vi "WT300 IEC 2015 Setup.vi"(0 "VISA Input":refnum<visa-resource-name>="WT210", 5 "Update Rate (250m s)":dbl(ring)=0.1 format="%#_13g" items=["100m"=0.1, "250m"=0.25, "500m"=0.5, "1"=1.0, "2"=2.0, "5"=5.0], 7 "Range Configuration (True)":bool[](array[boolean])=[FALSE, FALSE, FALSE, FALSE, FALSE, FALSE, FALSE, TRUE, TRUE, TRUE, TRUE, TRUE, FALSE], 11 "error in (no error)":errorcluster, 12 "Enable Auto Range (F: Disable)":bool, 13 "Manual Range (20 <10> A)":dbl(ring)=10.0 items=["5m <2.5m>"=0.0025, "10m <5m>"=0.005, "20m <10m>"=0.01, "50m <25m>"=0.025, "100m <50m>"=0.05, "200m <100m>"=0.1, "500m <250m>"=0.25, "1 <500m>"=0.5, "2 <1>"=1.0, "5 <2.5>"=2.5, "10 <5>"=5.0, "20 <10>"=10.0, "40 <20>"=20.0]) -> (2 "VTHD":sgl=0.065 format="%.3g", 4 "VISA Output":refnum<visa-resource-name>="WT210", 6 "Header File":string[][](array[string])=[["Instrument", "YOKOGAWA,WT332,C2QB17128V,F1.03\n"], ["Instr Driver Revision", "1.0 F1.03"], ["Start Time", "1.0"], ["Voltage Range", "6/1/2015 11:50 AM"], ["Current Range", "Auto"], ["Update Rate", "Auto"], ["Standard", "0.250"], ["Algorithm", "IEC62301 Ed.2(Auto)"], ["Stop Factor", "Linear Regression"], ["Valid Period", ""], ["Start Total Harmonic Distortion Uthd 1", "0.065"], ["Start Total Harmonic Distortion Uthd 2", ""], ["End Total Harmonic Distortion Uthd 1", ""], ["End Total Harmonic Distortion Uthd 2", ""], ["Max Power (Watts)", ""], ["Power Variation (%)", ""], ["", ""]], 15 "error out":errorcluster)   [LabVIEW 2016]
uses:
  <vilib>/Utility/error.llb/whitespace.ctl
  Public/Utility/Function/Create Function String (Harmonics).vi
  Public/Data/Read Measurement (Normal).vi
  Yokogawa WT300 Series.lvlib
panel:
  out "Date & Time":string="6/1/2015 11:50 AM"
  out "Instrument ID":string="YOKOGAWA,WT332,C2QB17128V,F1.03\n"
  out "Sample Rate":string="0.250"
  # "5m <2.5m> A"
  # "10m <5m> A"
  # "20m <10m> A"
  # "50m <25m> A"
  # "100m <50m> A"
  # "200m <100m> A"
  # "500m <250m> A"
  # "1 <500m> A"
  # "2 <1> A"
  # "5 <2.5> A"
  # "10 <5> A"
  # "20 <10> A"
  # "40 <20> A"
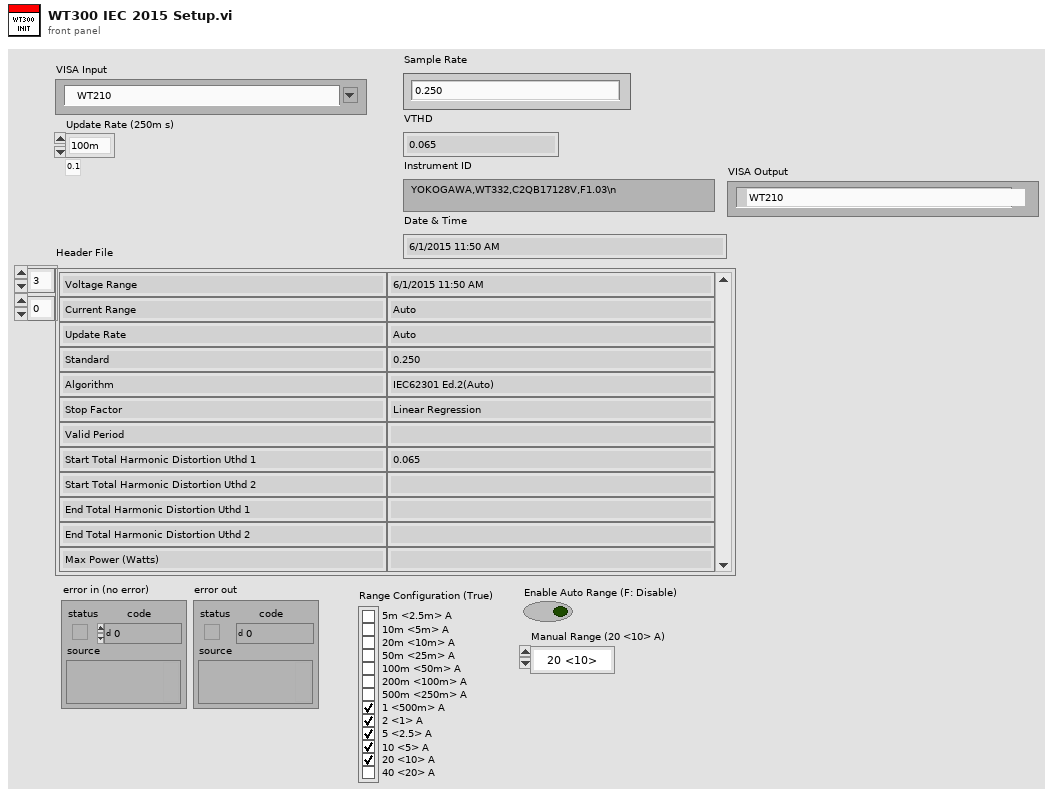
[diagram p1: front panel]
types:
  T1 = typedef "whitespace.ctl" = u16
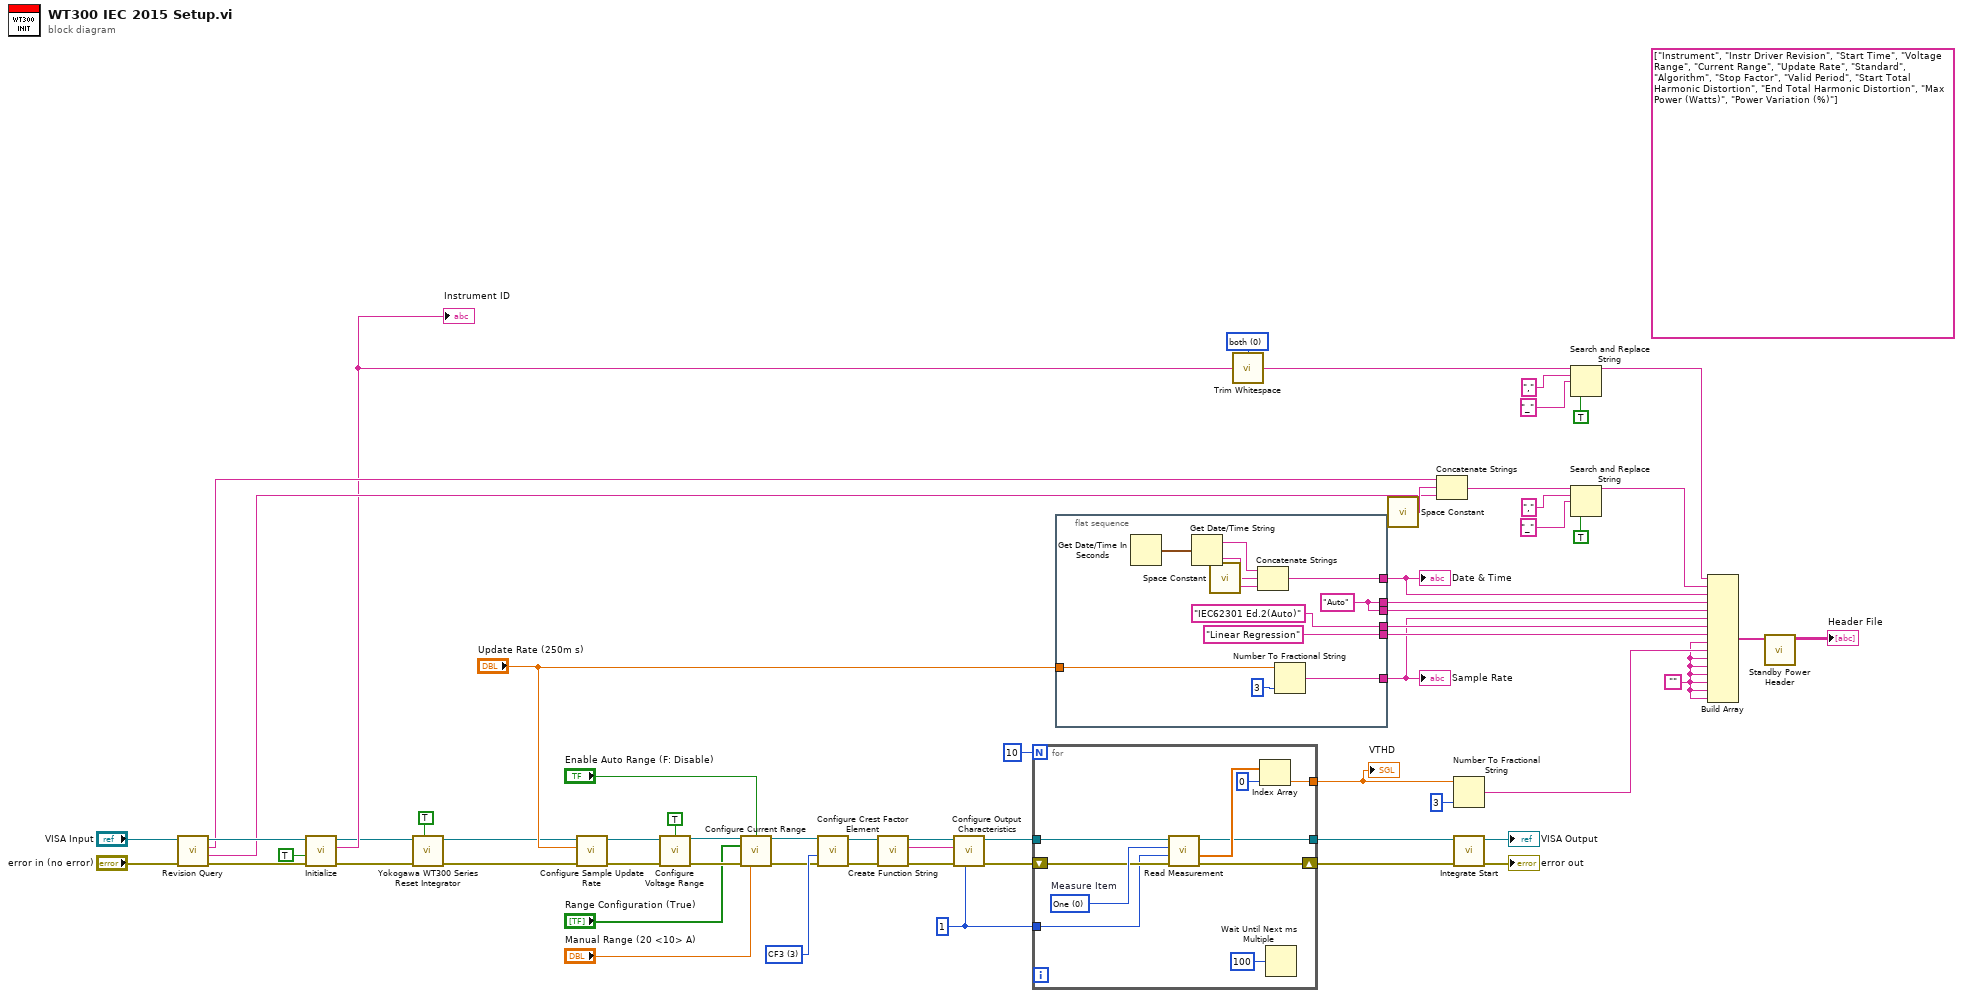
[diagram p0: block diagram]
diagram:
  w19 = T1 0 items=["both", "start of string", "end of string"] ("location (both)")
  w25 = 1 ("Item (1)")
  w41 = 3 items=["CF3"=3, "CF6"=6] ("Crest Factor (3: CF3)")
  w33 = ""
  (unwired) string[] ["Instrument", "Instr Driver Revision", "Start Time", "Voltage Range", "Current Range", "Update Rate", "Standard", "Algorithm", "Stop Factor", "Valid Period", "Start Total Harmonic Distortion", "End Total Harmonic Distortion", "Max Power (Watts)", "Power Variation (%)"]
  n1 = call "Revision Query.vi"("error in (no error)"="error in (no error)", "VISA resource name"="VISA Input") -> ("error out"=w49:errorcluster, "Instrument Firmware Revision"=w50:string, "Instrument Driver Revision"=w51:string, "VISA resource name out"=w52:refnum<visa-resource-name>)  [unwired: 6 in]
  n2 = call "Initialize.vi"("error in (no error)"=w49, "Reset (True)"=TRUE, "VISA resource name"=w52) -> ("error out"=w3:errorcluster, "Instrument ID"=w20:string, "VISA resource name out"=w4:refnum<visa-resource-name>)  [unwired: 6 in]
  "Instrument ID" <- w20
  n3 = call "Yokogawa WT300 Series Reset Integrator.vi"("Initialization Routing?"=TRUE, "Error In"=w3, "VISA Refnum in"=w4) -> ("Error Out"=w2:errorcluster, "VISA resource name out"=w1:refnum<visa-resource-name>)  [unwired: 7 in]
  n4 = call "Configure Sample Update Rate.vi"("error in (no error)"=w2, "Update Rate (500m s)"="Update Rate (250m s)", "VISA resource name"=w1) -> ("error out"=w48:errorcluster, "VISA resource name out"=w46:refnum<visa-resource-name>)  [unwired: 7 in]
  n5 = call "Configure Voltage Range.vi"("VISA resource name"=w46, "Enable Auto Range (F: Disable)"=TRUE, "error in (no error)"=w48) -> ("VISA resource name out"=w45:refnum<visa-resource-name>, "error out"=w44:errorcluster)  [unwired: 11 in]
  n6 = call "Configure Current Range.vi"("VISA resource name"=w45, "Enable Auto Range (F: Disable)"="Enable Auto Range (F: Disable)", "Range Configuration (True)"="Range Configuration (True)", "error in (no error)"=w44, "Manual Range (20 <10> A)"="Manual Range (20 <10> A)") -> ("VISA resource name out"=w39:refnum<visa-resource-name>, "error out"=w40:errorcluster)  [unwired: 9 in]
  n7 = call "Configure Crest Factor Element.vi"("error in (no error)"=w40, "Crest Factor (3: CF3)"=w41, "VISA resource name"=w39) -> ("error out"=w29:errorcluster, "VISA resource name out"=w28:refnum<visa-resource-name>)  [unwired: 7 in]
  n8 = call-poly "Create Function String.vi"("error in (no error)"=w29, "VISA resource name"=w28) -> ("error out"=w30:errorcluster, "Function String"=w31:string, "VISA resource name out"=w32:refnum<visa-resource-name>)  [unwired: 7 in]
  n9 = call "Configure Output Characteristics.vi"("Item (1)"=w25, "error in (no error)"=w30, "Function (Empty)"=w31, "VISA resource name"=w32) -> ("error out"=w26:errorcluster, "VISA resource name out"=w27:refnum<visa-resource-name>)  [unwired: 6 in]
  n10 = for {
    N: 10 -> [_]
    tunnel: w27 -> [w69]
    tunnel: w25 -> [w67]
    tunnel: [w65] -> w22
    tunnel: [w64] -> w36
    shift-right: [w66] -> w23
    shift-left: w26 -> [w68]
    w70 = 0 items=["One", "Plural"]  # Measure Item
    n11 = call-poly "Read Measurement.vi"("error in (no error)"=w68, "Number of Item (15)"=w67, "Measure Item (1: Plural)"=w70, "VISA resource name"=w69) -> ("error out"=w66:errorcluster, "Measurement"=w71:dbl[], "VISA resource name out"=w65:refnum<visa-resource-name>)  [unwired: 4 in, 1 out]
    n12 = Index Array(array=w71, index=0 ("指標 （行）")) -> (element=w64:dbl)
    n13 = Wait Until Next ms Multiple(millisecond multiple=u32 100) -> ()  [unwired: 1 out]
  }
  "VTHD" <- w36
  n14 = flat-sequence {
    tunnel: [w76] -> w62
    tunnel: [w76] -> w61
    tunnel: ["IEC62301 Ed.2(Auto)" ("element")] -> w60
    tunnel: ["Linear Regression" ("element")] -> w59
    tunnel: [w77] -> w56
    tunnel: [w75] -> w55
    tunnel: "Update Rate (250m s)" -> [w74]
    frame #0 {
      w76 = "Auto"
      n15 = Get Date/Time In Seconds() -> (seconds since 1Jan1904=w78:timestamp)
      n16 = Get Date/Time String(seconds (now)=w78) -> (date string=w80:string, time string=w81:string)  [unwired: 2 in]
      n17 = call <vilib>:"Space Constant.vi"() -> ("String"=w79:string)
      n18 = Concatenate Strings(w80, w79, w81) -> (w77:string)
      n19 = Number To Fractional String(number=w74, precision (6)=i16 3) -> (F-format string=w75:string)  [unwired: 2 in]
    }
  }
  n20 = call <vilib>:"Trim Whitespace.vi"("string"=w20, "location (both)"=w19) -> ("trimmed string"=w9:string)
  n21 = call <vilib>:"Space Constant.vi"() -> ("String"=w57:string)
  n22 = Concatenate Strings(w51, w57, w50) -> (w14:string)
  n23 = Number To Fractional String(number=w36, precision (6)=i16 3) -> (F-format string=w34:string)  [unwired: 2 in]
  n24 = call "Integrate Start.vi"("error in (no error)"=w23, "VISA resource name"=w22) -> ("error out"=→"error out":errorcluster, "VISA resource name out"=→"VISA Output":refnum<visa-resource-name>)  [unwired: 8 in]
  n25 = Search and Replace String(replace all?=TRUE ("replace all? (F)"), input string=w9, search string=",", replace string="_" ("replace string (\"\")")) -> (result string=w8:string)  [unwired: 4 in, 3 out]
  n26 = Search and Replace String(replace all?=TRUE ("replace all? (F)"), input string=w14, search string=",", replace string="_" ("replace string (\"\")")) -> (result string=w13:string)  [unwired: 4 in, 3 out]
  n27 = Build Array(w8, w13, w56, w62, w61, w55, w60, w59, w33, w34, w33, w33, w33, w33, w33, w33) -> (w58:string[])
  n28 = call "Standby Power Header.vi"("Array"=w58) -> ("Header File"=→"Header File":string[][])  [unwired: 9 in, 1 out]
  "Sample Rate" <- w55
  "Date & Time" <- w56
